vi "target run 2.vi"() -> ()   [LabVIEW 2012]
uses:
  <vilib>/robotics/Starter Kit/2.0/9632 Host Interface/NI_Robotics_Starter Kit Host_9632_2.0.lvclass
  <vilib>/robotics/Starter Kit/Host Interface/NI_Robotics_Starter Kit Host.lvclass
panel:
  out "Waveform Chart 2":cluster{dbl, dbl}(graph)
  out "Waveform Chart":cluster{"distance 2":dbl, dbl}(graph)
  out "CF":dbl
  out "Beta (rad)":dbl
  out "F_1A_1":dbl
  out "A_1B_1":dbl
  out "A_1F":dbl
  out "s":dbl
  in  "stop":bool
  out "F_1B_1":dbl
  out "cos_2alpha":dbl
  out "Beta (deg)":dbl
  in  "distance 2":dbl
  out "MF":dbl
  out "gamma (rad)":dbl
  out "gamma (deg)":dbl
  out "MC":dbl
  in  "k_2":dbl
  in  "k_1":dbl
  in  "k":dbl
  out "V_Mx":dbl
  out "V_My":dbl
  out "MC_x":dbl
  out "MC_y":dbl
  out "distance":dbl
  out "MC_xi":dbl
  out "MC_yi":dbl
  out "w_L":dbl
  out "w_R":dbl
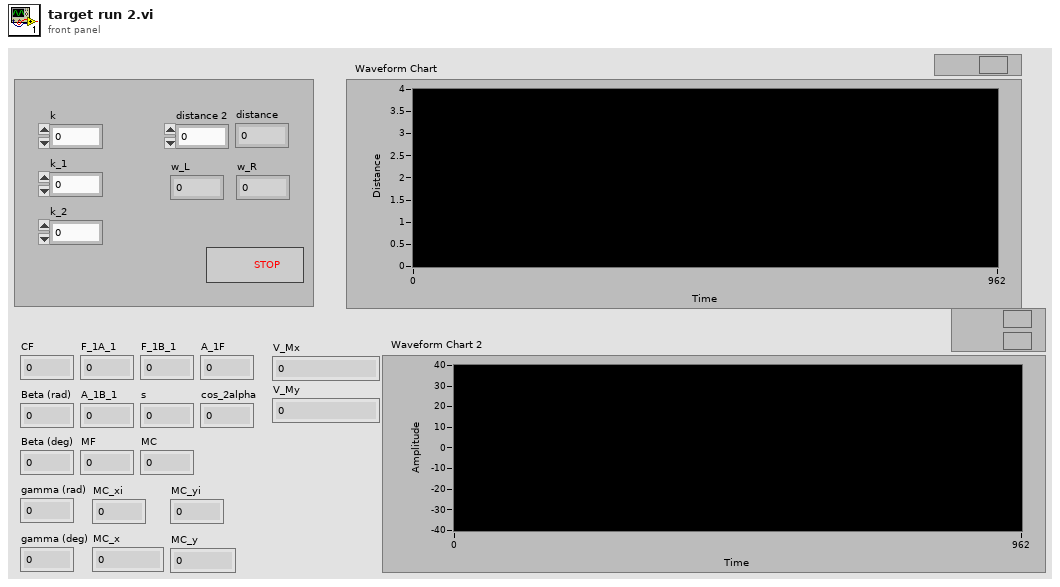
[diagram p1: front panel]
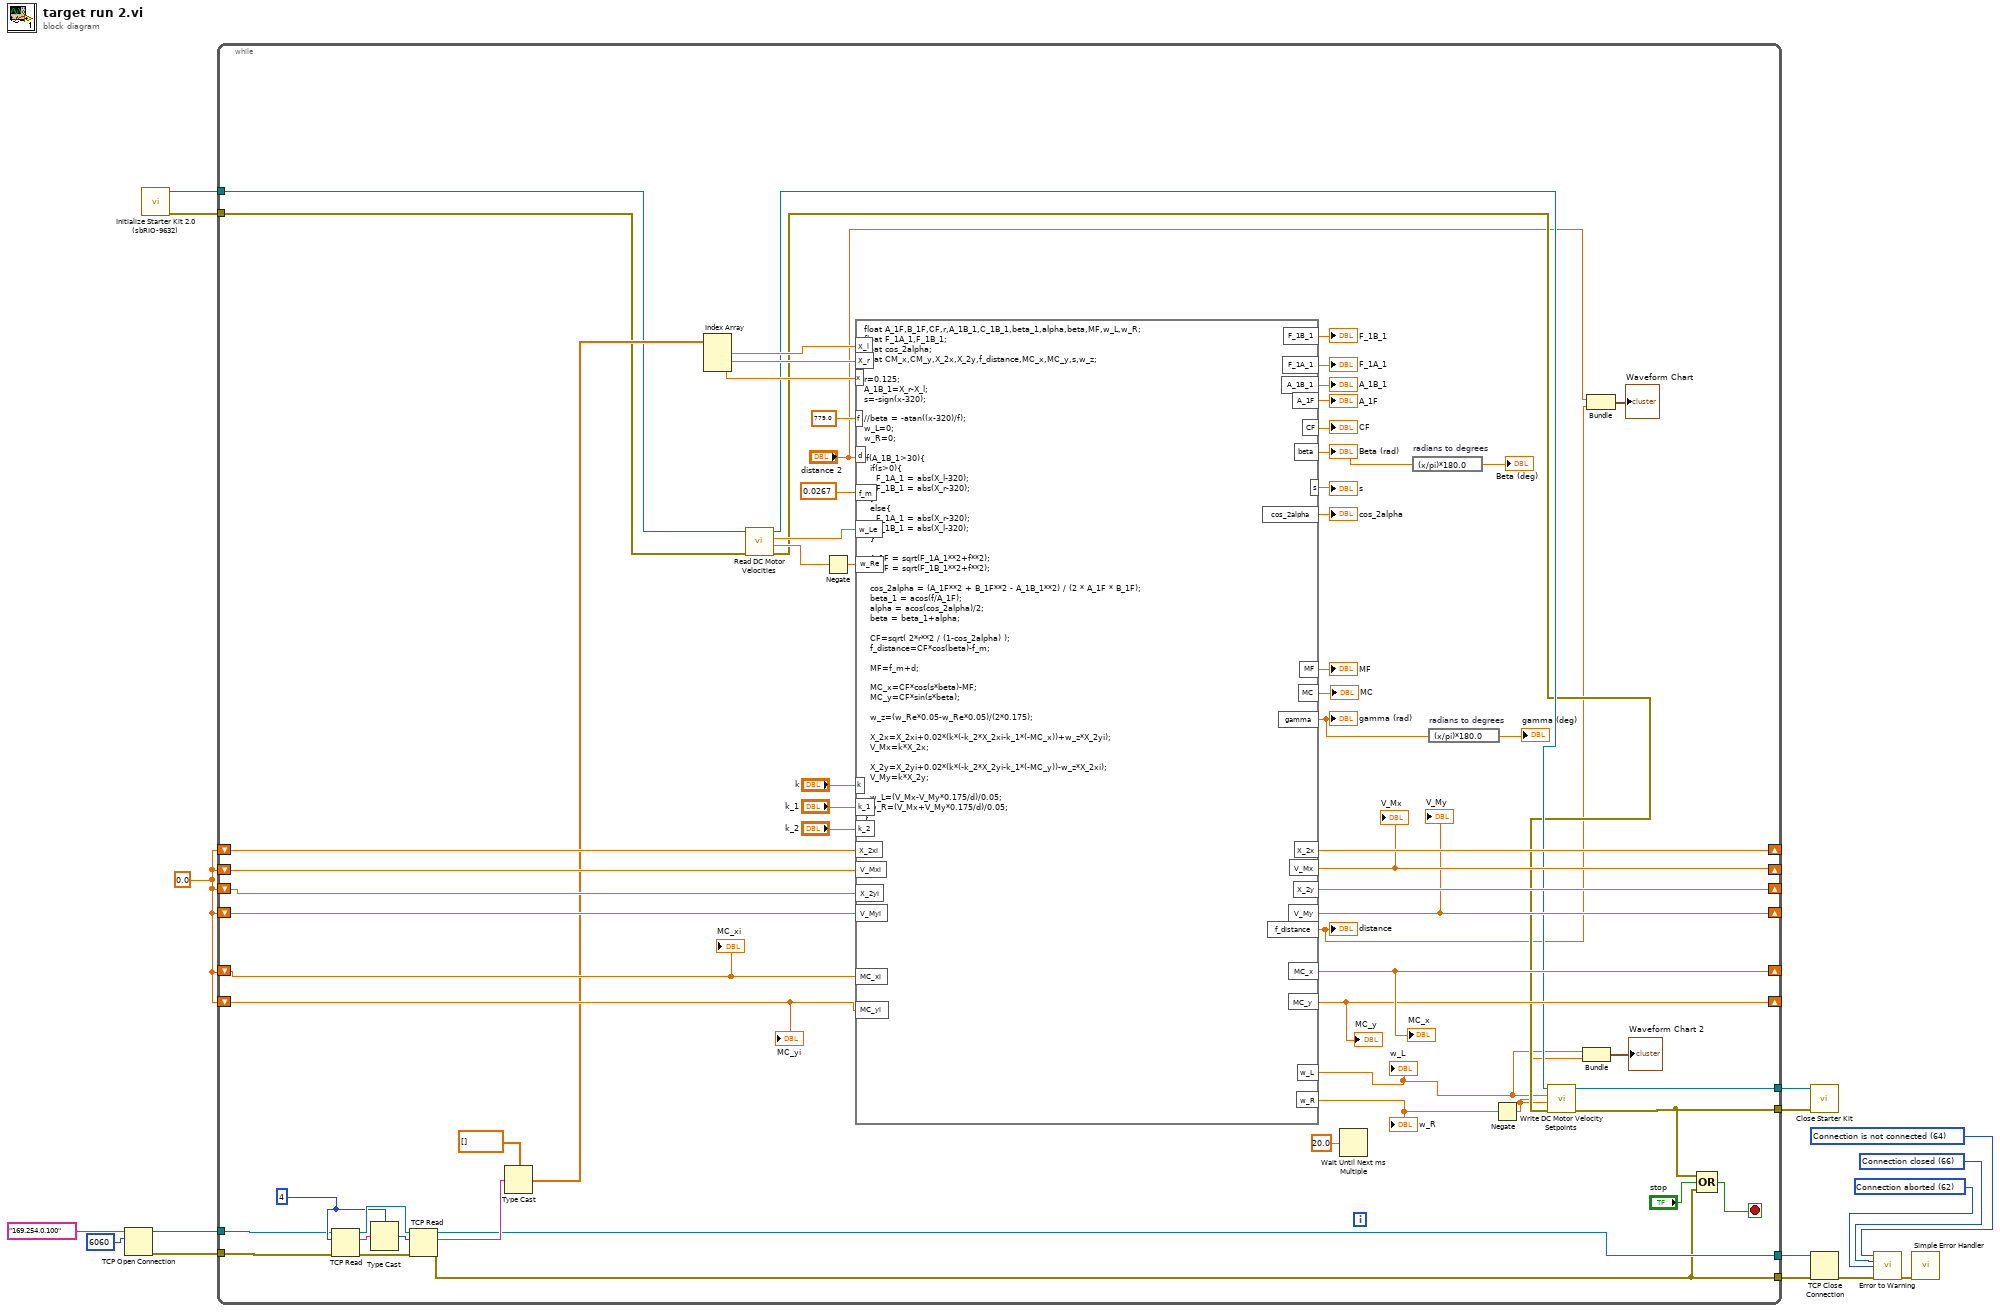
[diagram p0: block diagram]
diagram:
  w3 = 62 items=["No Error", "Argument Error", "Memory Full", "Out of Zone", "End of File", "File Already Open", "Generic File IO Error", "File Not Found", "File Permission Error", "Disk Full", "Duplicate Path", "Too Many Files Open", "Not Enabled", "Resource File Not Found", "Cannot Add Resource", "Resource Not Found", "Image Not Found", "Image Memory Error", "Pen Does Not Exist", "Config Bad Type", "Config Token Not Found", "Config Parse Error", "Config Memory Error", "Bad External Code Format", "Bad External Code Offset", "External Code Not Present", "Null Window", "Destroy Window Mixup", "Null Menu", "Print Aborted", "Bad Print Record", "Print Driver Error", "Windows Error During Print", "Memory Error During Print", "Print Dialog Error", "Generic Print Error", "Invalid Device Refnum", "Device Not Found", "Device Parameter Error", "Device Unit Error", "Can't Open Device", "Device Call Aborted", "Generic Error", "Cancelled By User", "Object ID Too Low", "Object ID Too High", "Object Not In Heap", "Unknown Heap", "Bad DefProc ID", "DefProc Not In Table", "Message Out Of Range", "Null Method", "Unknown Message", "Manager Call Not Supported", "Bad address", "Connection In progress", "Connection timed out", "Connection is already in progress", "Network attribute not supported", "Network error", "Address in use", "System out of memory", "Connection aborted", "Connection refused", "Connection is not connected", "Connection is already connected", "Connection closed", "Initialize error (interapplication manager)", "Bad occurrence", "Wait on unbound occurrence handler", "Occurrence queue overflow", "Bad path", "Semaphore not signaled", "Unrecognized type (interapplication manager)"] ("1st Error to Convert")
  w2 = 66 items=["No Error", "Argument Error", "Memory Full", "Out of Zone", "End of File", "File Already Open", "Generic File IO Error", "File Not Found", "File Permission Error", "Disk Full", "Duplicate Path", "Too Many Files Open", "Not Enabled", "Resource File Not Found", "Cannot Add Resource", "Resource Not Found", "Image Not Found", "Image Memory Error", "Pen Does Not Exist", "Config Bad Type", "Config Token Not Found", "Config Parse Error", "Config Memory Error", "Bad External Code Format", "Bad External Code Offset", "External Code Not Present", "Null Window", "Destroy Window Mixup", "Null Menu", "Print Aborted", "Bad Print Record", "Print Driver Error", "Windows Error During Print", "Memory Error During Print", "Print Dialog Error", "Generic Print Error", "Invalid Device Refnum", "Device Not Found", "Device Parameter Error", "Device Unit Error", "Can't Open Device", "Device Call Aborted", "Generic Error", "Cancelled By User", "Object ID Too Low", "Object ID Too High", "Object Not In Heap", "Unknown Heap", "Bad DefProc ID", "DefProc Not In Table", "Message Out Of Range", "Null Method", "Unknown Message", "Manager Call Not Supported", "Bad address", "Connection In progress", "Connection timed out", "Connection is already in progress", "Network attribute not supported", "Network error", "Address in use", "System out of memory", "Connection aborted", "Connection refused", "Connection is not connected", "Connection is already connected", "Connection closed", "Initialize error (interapplication manager)", "Bad occurrence", "Wait on unbound occurrence handler", "Occurrence queue overflow", "Bad path", "Semaphore not signaled", "Unrecognized type (interapplication manager)"] ("1st Error to Convert")
  w1 = 64 items=["No Error", "Argument Error", "Memory Full", "Out of Zone", "End of File", "File Already Open", "Generic File IO Error", "File Not Found", "File Permission Error", "Disk Full", "Duplicate Path", "Too Many Files Open", "Not Enabled", "Resource File Not Found", "Cannot Add Resource", "Resource Not Found", "Image Not Found", "Image Memory Error", "Pen Does Not Exist", "Config Bad Type", "Config Token Not Found", "Config Parse Error", "Config Memory Error", "Bad External Code Format", "Bad External Code Offset", "External Code Not Present", "Null Window", "Destroy Window Mixup", "Null Menu", "Print Aborted", "Bad Print Record", "Print Driver Error", "Windows Error During Print", "Memory Error During Print", "Print Dialog Error", "Generic Print Error", "Invalid Device Refnum", "Device Not Found", "Device Parameter Error", "Device Unit Error", "Can't Open Device", "Device Call Aborted", "Generic Error", "Cancelled By User", "Object ID Too Low", "Object ID Too High", "Object Not In Heap", "Unknown Heap", "Bad DefProc ID", "DefProc Not In Table", "Message Out Of Range", "Null Method", "Unknown Message", "Manager Call Not Supported", "Bad address", "Connection In progress", "Connection timed out", "Connection is already in progress", "Network attribute not supported", "Network error", "Address in use", "System out of memory", "Connection aborted", "Connection refused", "Connection is not connected", "Connection is already connected", "Connection closed", "Initialize error (interapplication manager)", "Bad occurrence", "Wait on unbound occurrence handler", "Occurrence queue overflow", "Bad path", "Semaphore not signaled", "Unrecognized type (interapplication manager)"] ("1st Error to Convert")
  w16 = 0.0 ("V_My")
  n1 = TCP Open Connection(address="169.254.0.100", remote port or service name=u16 6060) -> (connection ID=w13:refnum<k5>, error out=w12:errorcluster)  [unwired: 3 in]
  n2 = call <vilib>:"Initialize Starter Kit 2.0 (sbRIO-9632).vi"() -> ("error out"=w8:errorcluster, "FPGA starter kit host 2.0 out"=w9:refnum<class "NI_Robotics_Starter Kit Host_9632_2.0.lvclass">)  [unwired: 10 in]
  n3 = while {
    shift-right: [w62] -> _
    shift-left: w16 -> [w61]
    shift-right: [w63] -> _
    shift-left: w16 -> [w59]
    shift-right: [w64] -> _
    shift-left: w16 -> [w60]
    shift-right: [w65] -> _
    shift-left: w16 -> [w58]
    shift-right: [w53] -> _
    shift-left: w16 -> [w55]
    shift-right: [w52] -> _
    shift-left: w16 -> [w54]
    tunnel: w13 -> [w42]
    tunnel: w12 -> [w43]
    tunnel: [w26] -> w11
    tunnel: [w41] -> w10
    tunnel: w9 -> [w32]
    tunnel: w8 -> [w30]
    tunnel: [w36] -> w7
    tunnel: [w28] -> w6
    stop <- w25 stop-if-true
    w44 = 4 ("bytes to read")
    n4 = TCP Read(connection ID=w42, bytes to read=w44, error in (no error)=w43) -> (connection ID out=w48:refnum<k5>, data out=w47:string, error out=w49:errorcluster)  [unwired: 2 in]
    n5 = Type Cast(type=w44, x=w47) -> (*(type *) &x=w50:i32)
    n6 = TCP Read(connection ID=w48, bytes to read=w50, error in (no error)=w49) -> (connection ID out=w41:refnum<k5>, data out=w45:string, error out=w26:errorcluster)  [unwired: 2 in]
    n7 = Type Cast(type=dbl[] [] ("appended array"), x=w45) -> (*(type *) &x=w46:dbl[])
    n8 = Index Array(array=w46) -> (element #1=w39:dbl, element #2=w38:dbl, element #3=w37:dbl)  [unwired: 3 in]
    n9 = call <vilib>:"Read DC Motor Velocities.vi"("error in (no error)"=w30, "starter kit host in"=w32) -> ("error out"=w29:errorcluster, "right motor ccw velocity (rad/s)"=w33:dbl, "left motor ccw velocity (rad/s)"=w35:dbl, "starter kit host out"=w31:refnum<class "NI_Robotics_Starter Kit Host_9632_2.0.lvclass">)  [unwired: 6 in]
    n10 = Negate(x=w33) -> (-x=w34:dbl)
    n11 = formula code="float A_1F,B_1F,CF,r,A_1B_1,C_1B_1,beta_1,alpha,beta,MF,w_L,w_R;\nfloat F_1A_1,F_1B_1;\nfloat cos_2alpha;\nfloat CM_x,CM_y,X_2x,X_2y,f_distance,MC_x,MC_y,s,w_z;\n\nr=0.125;\nA_1B_1=X_r-X_l;\ns=-sign(x-320);\n\n//beta = -atan((x-320)/f);\nw_L=0;\nw_R=0;\n\nif(A_1B_1>30){  \n  if(s>0){\n    F_1A_1 = abs(X_l-320);\n    F_1B_1 = abs(X_r-320);\n  }\n  else{\n    F_1A_1 = abs(X_r-320);\n    F_1B_1 = abs(X_l-320);\n  }\n\n  A_1F = sqrt(F_1A_1**2+f**2);\n  B_1F = sqrt(F_1B_1**2+f**2);\n \n  cos_2alpha = (A_1F**2 + B_1F**2 - A_1B_1**2) / (2 * A_1F * B_1F);\n  beta_1 = acos(f/A_1F);\n  alpha = acos(cos_2alpha)/2;\n  beta = beta_1+alpha;\n\n  CF=sqrt( 2*r**2 / (1-cos_2alpha) );\n  f_distance=CF*cos(beta)-f_m;\n\n  MF=f_m+d;\n\n  MC_x=CF*cos(s*beta)-MF;\n  MC_y=CF*sin(s*beta);\n   \n  w_z=(w_Re*0.05-w_Re*0.05)/(2*0.175);\n\n  X_2x=X_2xi+0.02*(k*(-k_2*X_2xi-k_1*(-MC_x))+w_z*X_2yi);\n  V_Mx=k*X_2x;\n\n  X_2y=X_2yi+0.02*(k*(-k_2*X_2yi-k_1*(-MC_y))-w_z*X_2xi);\n  V_My=k*X_2y;\n\n  w_L=(V_Mx-V_My*0.175/d)/0.05;\n  w_R=(V_Mx+V_My*0.175/d)/0.05;\n}"("X_l"=w39, "X_r"=w38, "x"=w37, "f"=779.0 ("input variable"), "d"="distance 2", "f_m"=0.0267 ("input variable"), "X_2yi"=w60, "X_2xi"=w58, "V_Mxi"=w59, "V_Myi"=w61, "k_2"="k_2", "k_1"="k_1", "k"="k", "MC_xi"=w55, "MC_yi"=w54, "w_Re"=w34, "w_Le"=w35) -> ("CF"=→"CF":dbl, "beta"=w73:dbl, "F_1A_1"=→"F_1A_1":dbl, "A_1B_1"=→"A_1B_1":dbl, "A_1F"=→"A_1F":dbl, "s"=→"s":dbl, "F_1B_1"=→"F_1B_1":dbl, "cos_2alpha"=→"cos_2alpha":dbl, "MF"=→"MF":dbl, "gamma"=w69:dbl, "MC"=→"MC":dbl, "X_2x"=w65:dbl, "X_2y"=w64:dbl, "V_Mx"=w63:dbl, "V_My"=w62:dbl, "f_distance"=w19:dbl, "MC_x"=w53:dbl, "MC_y"=w52:dbl, "w_L"=w18:dbl, "w_R"=w17:dbl)
    "Beta (rad)" <- w73
    "gamma (rad)" <- w69
    "V_Mx" <- w63
    "V_My" <- w62
    "MC_x" <- w53
    "MC_y" <- w52
    "distance" <- w19
    "w_L" <- w18
    "w_R" <- w17
    n12 = Wait Until Next ms Multiple(millisecond multiple=20.0) -> ()  [unwired: 1 out]
    n13 = expression code="(x/pi)*180.0" "radians to degrees"(w73) -> (→"Beta (deg)":dbl)
    n14 = expression code="(x/pi)*180.0" "radians to degrees"(w69) -> (→"gamma (deg)":dbl)
    n15 = Negate(x=w17) -> (-x=w22:dbl)
    n16 = call <vilib>:"Write DC Motor Velocity Setpoints.vi"("error in (no error)"=w29, "right motor ccw velocity (rad/s)"=w22, "left motor ccw velocity (rad/s)"=w18, "starter kit host in"=w31) -> ("error out"=w28:errorcluster, "starter kit host out"=w36:refnum<class "NI_Robotics_Starter Kit Host_9632_2.0.lvclass">)  [unwired: 6 in]
    n17 = Bundle(w18, w22) -> (→"Waveform Chart 2":cluster{dbl, dbl})  [unwired: 1 in]
    n18 = Bundle("distance 2"="distance 2", w19) -> (→"Waveform Chart":cluster{"distance 2":dbl, dbl})  [unwired: 1 in]
    n19 = Compound Arithmetic op=OR(w28, "stop", w26) -> (w25:bool)
    "MC_xi" <- w55
    "MC_yi" <- w54
  }
  n20 = call-dynamic "Close Starter Kit.vi"("error in (no error)"=w6, "starter kit host in"=w7) -> ()  [unwired: 9 in, 1 out]
  n21 = TCP Close Connection(connection ID=w10, error in (no error)=w11) -> (error out=w4:errorcluster)  [unwired: 1 in, 1 out]
  n22 = call <vilib>:"Error to Warning.vi"("1st Error to Convert"=w1, "2nd Error to Convert"=w2, "3rd Error to Convert"=w3, "error in"=w4) -> ("warning out"=w5:errorcluster)  [unwired: 11 in]
  n23 = call <vilib>:"Simple Error Handler.vi"("error in (no error)"=w5) -> ()  [unwired: 4 in, 5 out]
